vi "Read Connections.vi"(8 "error in (no error)":errorcluster, 11 "Mock %DEVICE% Consumer in":refnum<class "Mock %DEVICE% Consumer.lvclass">) -> (0 "error out":errorcluster, 2 "Connections":string[](array[string]), 3 "Mock %DEVICE% Consumer out":refnum<class "Mock %DEVICE% Consumer.lvclass">)   [LabVIEW 2017, in "Mock %DEVICE% Consumer.lvclass"]
uses:
  Mock %DEVICE% Consumer.lvclass
  Mock %DEVICE% Consumer.lvclass/Mock %DEVICE% Consumer.ctl
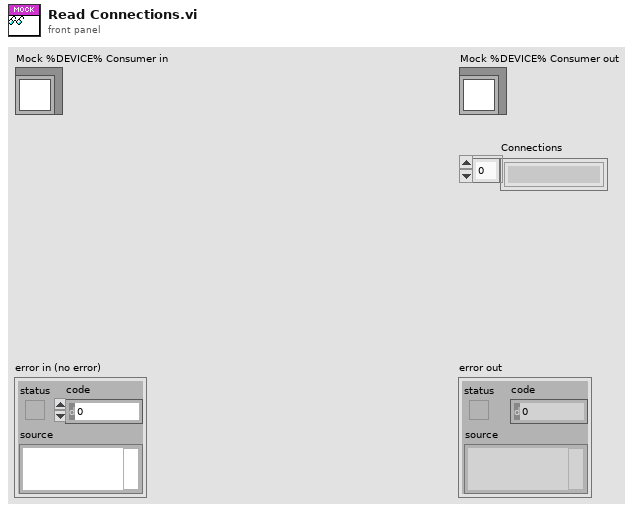
[diagram p1: front panel]
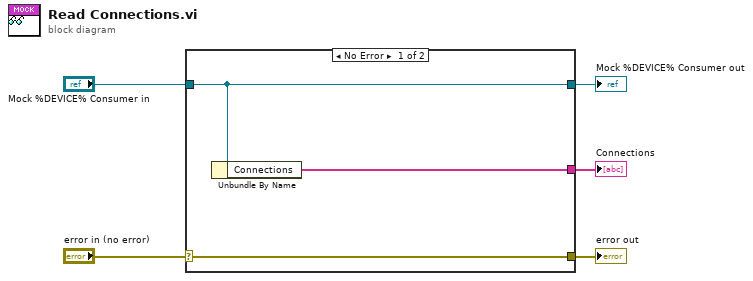
[diagram p0: block diagram]
diagram:
  n1 = case shown="No Error" "error in (no error)" {
    selector: "error in (no error)" -> [w8 w9]
    tunnel: [w8 w9] -> w4
    tunnel: [w7 w10] -> w2
    tunnel: "Mock %DEVICE% Consumer in" -> [w7 w10]
    tunnel: [w6 _] -> w1
    frame No Error {
      n2 = Unbundle By Name(w7) -> ("Connections"=w6:string[])
    }
    frame Error {
    }
  }
  "error out" <- w4
  "Mock %DEVICE% Consumer out" <- w2
  "Connections" <- w1
